vi "Pololu.Mgr - Set All to OFF.vi"(8 "error in (no error)":errorcluster, 11 "PololuCtrl in":refnum<class "PololuCtrl.lvclass">) -> (0 "error out":errorcluster, 3 "PololuCtrl out":refnum<class "PololuCtrl.lvclass">)   [LabVIEW 2018, in "PololuCtrl.lvclass"]
uses:
  PololuCtrl.lvclass
  PololuCtrl.lvclass/PololuCtrl.ctl
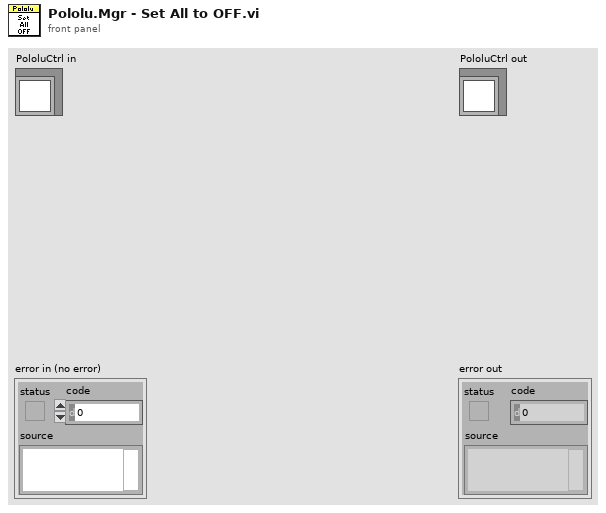
[diagram p1: front panel]
types:
  T1 = typedef "Pololu.Device Config.ctl" = cluster{"Chan":u8, "Accel":u16, "Speed":u16, "Positions":dbl[], "Range Info":T2}
  T2 = typedef "Pololu.Device Range Config.ctl" = cluster{"Min us":dbl, "Max us":dbl, "Min deg":dbl, "Max deg":dbl, "LStopDeg":dbl, "UStopDeg":dbl}
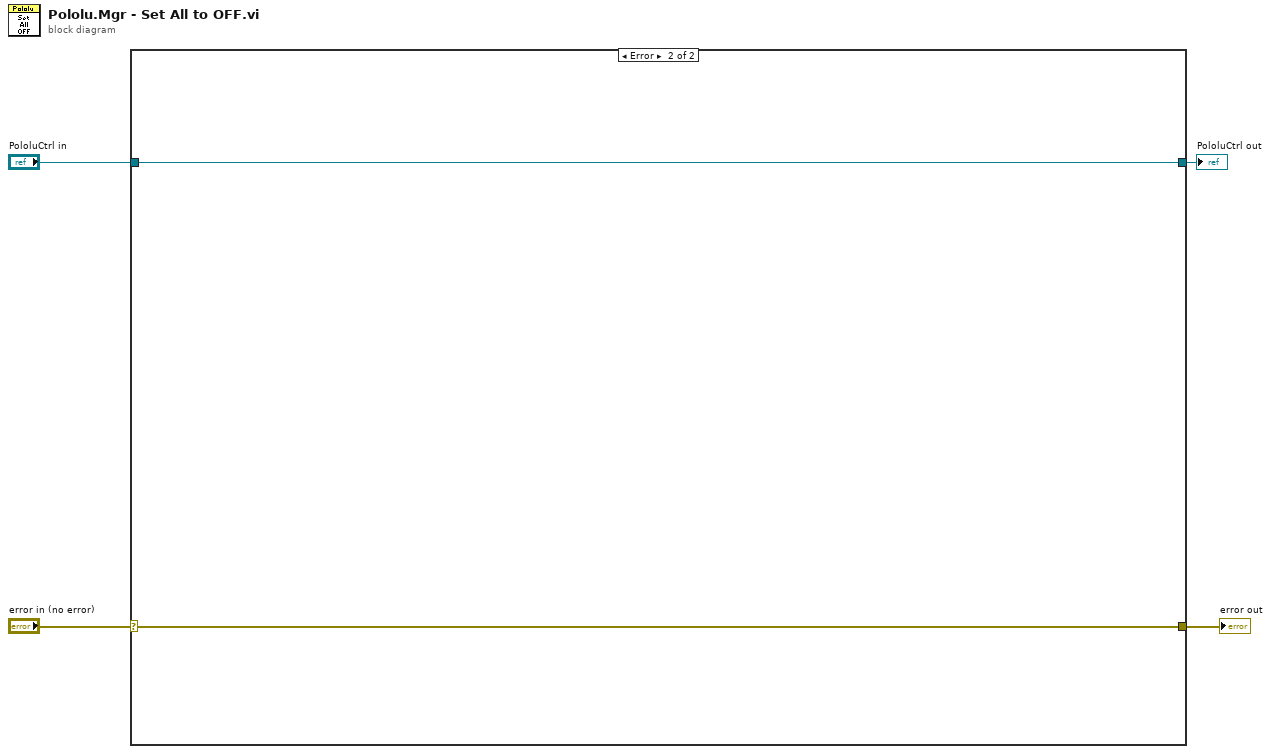
[diagram p0: block diagram]
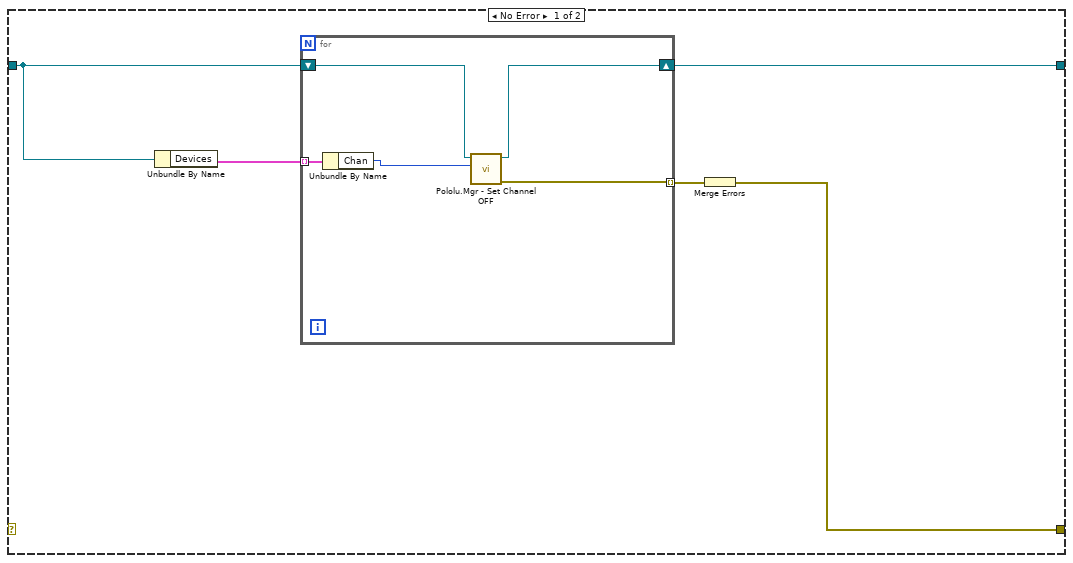
[diagram p2: hidden frame]
diagram:
  n1 = case shown="Error" "error in (no error)" {
    selector: "error in (no error)" -> [_ w16]
    tunnel: [w5 w16] -> w3
    tunnel: [w7 w15] -> w1
    tunnel: "PololuCtrl in" -> [w9 w15]
    frame No Error {
      n2 = Unbundle By Name(w9) -> ("Devices"=w8:T1[])
      n3 = for {
        tunnel: w8 -> [w13] mode=indexing
        tunnel: [w11] -> w6 mode=indexing
        shift-right: [w10] -> w7
        shift-left: w9 -> [w14]
        n4 = Unbundle By Name(w13) -> ("Chan"=w12:u8)
        n5 = call "Pololu.Mgr - Set Channel OFF.vi"("Channel"=w12, "PololuCtrl in"=w14) -> ("error out"=w11:errorcluster, "PololuCtrl out"=w10:refnum<class "PololuCtrl.lvclass">)  [unwired: 8 in]
      }
      n6 = Merge Errors(w6) -> (w5:errorcluster)
    }
    frame Error {
    }
  }
  "error out" <- w3
  "PololuCtrl out" <- w1
